vi "Get Control Size.vi"(8 "error in (no error)":errorcluster, 11 "Ctl Refnum":refnum<vi>) -> (0 "error out":errorcluster, 1 "Availible?":bool, 2 "Size":T1, 3 "refnum dub":refnum<vi>)   [LabVIEW 2014, in "POLARIS Vision utility.lvlib"]
uses:
  POLARIS Vision utility.lvlib
  <vilib>/Utility/miscctls.llb/LVBoundsTypeDef.ctl
  XDisplay/POLARIS IMAQ Display.xctl
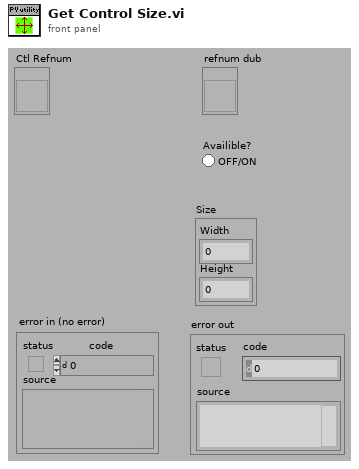
[diagram p1: front panel]
types:
  T1 = typedef "LVBoundsTypeDef.ctl" = cluster{"Width":u32, "Height":u32}
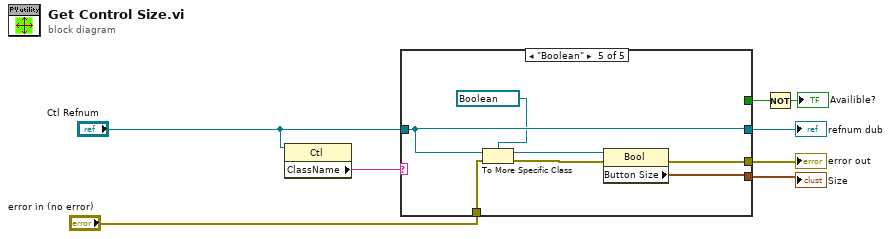
[diagram p0: block diagram]
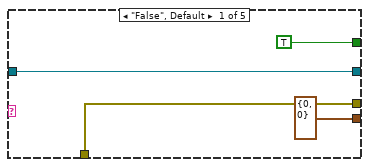
[diagram p2: hidden frame]
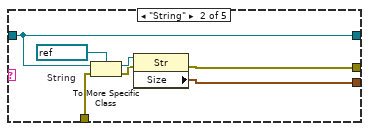
[diagram p3: hidden frame]
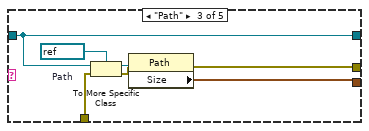
[diagram p4: hidden frame]
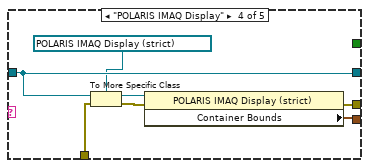
[diagram p5: hidden frame]
diagram:
  n1 = property class="Ctl"(reference="Ctl Refnum") -> ("ClassName"=w1:string)  [unwired: 1 in, 2 out]
  n2 = case shown="\"Boolean\"" w1 {
    tunnel: [w12 w14 w21 w32 w36] -> w8
    tunnel: "Ctl Refnum" -> [w12 w14 w21 w32 w36]
    tunnel: "error in (no error)" -> [w11 w17 w24 w31 w39]
    tunnel: [w11 w15 w22 w29 w37] -> w6
    tunnel: [TRUE _ _ _ _] -> w5
    tunnel: [T1 {"Width"=0, "Height"=0} ("Button Size") w13 w20 w27 w35] -> w3
    frame "False", Default {
    }
    frame "String" {
      w18 = refnum<vi> refnum  # String
      n3 = To More Specific Class(target class=w18, reference=w14, error in=w17) -> (specific class reference=w19:refnum<vi>, error out=w16:errorcluster)
      n4 = property class="Str"(reference=w19, error in=w16) -> (error out=w15:errorcluster, "Size"=w13:T1)  [unwired: 1 out]
    }
    frame "Path" {
      w25 = refnum<vi> refnum  # Path
      n5 = To More Specific Class(target class=w25, reference=w21, error in=w24) -> (specific class reference=w26:refnum<vi>, error out=w23:errorcluster)
      n6 = property class="Path"(reference=w26, error in=w23) -> (error out=w22:errorcluster, "Size"=w20:T1)  [unwired: 1 out]
    }
    frame "POLARIS IMAQ Display" {
      n7 = To More Specific Class(target class=refnum<vi> refnum ("POLARIS IMAQ"), reference=w32, error in=w31) -> (specific class reference=w33:refnum<vi>, error out=w30:errorcluster)
      n8 = property class="POLARIS IMAQ Display (strict)"(reference=w33, error in=w30) -> (error out=w29:errorcluster, "Container Bounds"=w27:T1)  [unwired: 1 out]
    }
    frame "Boolean" {
      n9 = To More Specific Class(target class=refnum<vi> refnum ("Bool Refnum"), reference=w36, error in=w39) -> (specific class reference=w40:refnum<vi>, error out=w38:errorcluster)
      n10 = property class="Bool"(reference=w40, error in=w38) -> (error out=w37:errorcluster, "Button Size"=w35:T1)  [unwired: 1 out]
    }
  }
  "refnum dub" <- w8
  "error out" <- w6
  "Size" <- w3
  n11 = Not(x=w5) -> (.not. x?=→"Availible?":bool)
